vi "TSCAN_GetDllPath.vi"() -> (3 "DllPath":path)   [LabVIEW 2014]
uses:
  Utilities/Global/DLL_Path.vi
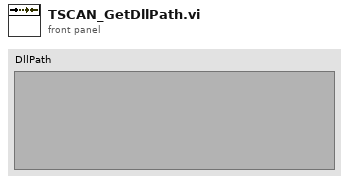
[diagram p1: front panel]
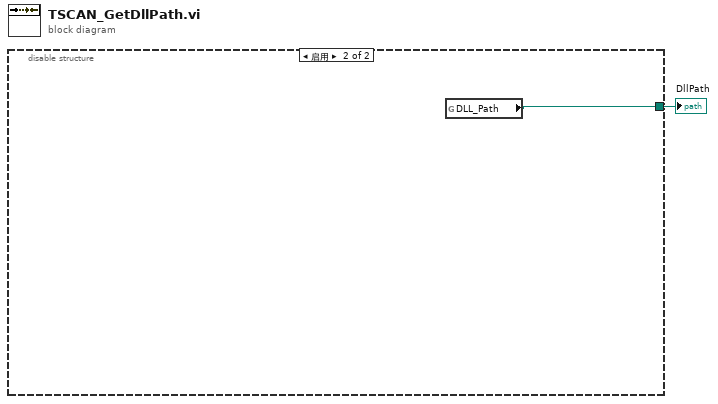
[diagram p0: block diagram]
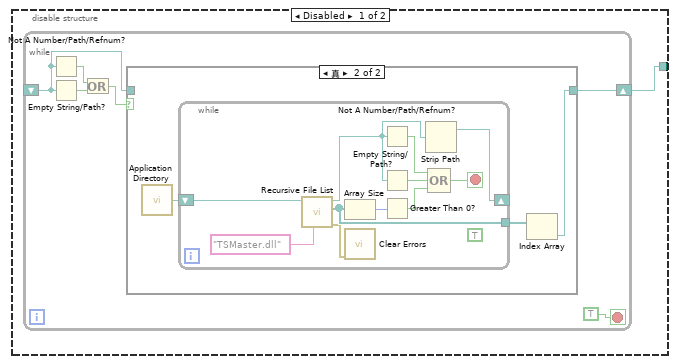
[diagram p2: hidden frame]
diagram:
  n1 = disable-structure shown="启用" {
    disable-tunnel: [w2 w24] -> w1
    frame Disabled {
      n2 = while {
        shift-right: [w8] -> w2
        shift-left: _ -> [w3]
        stop <- TRUE stop-if-true
        n3 = Not A Number/Path/Refnum?(number/path/refnum=w3) -> (NaN/Path/Refnum?=w6:bool)
        n4 = Empty String/Path?(string/path=w3) -> (empty?=w5:bool)
        n5 = Or(x=w6, y=w5) -> (x .or. y?=w4:bool)
        n6 = case shown="真" w4 {
          tunnel: [w9 w12] -> w8
          tunnel: w3 -> [w9 _]
          frame False {
          }
          frame True {
            n7 = call <vilib>:"Application Directory.vi"() -> ("Application Directory"=w10:path)
            n8 = while {
              shift-right: [w15] -> _
              shift-left: w10 -> [w23]
              tunnel: [w14] -> w11
              stop <- w17 stop-if-true
              (unwired) TRUE ("Treat LLBs as Folders?")
              n9 = call <vilib>:"Recursive File List.vi"("pattern"="TSMaster.dll", "Folder Path"=w23) -> ("error out"=w13:errorcluster, "All Files in Dir"=w14:path[], "dup Folder Path"=w16:path)  [unwired: 3 in, 4 out]
              n10 = Array Size(array=w14) -> (size(s)=w21:i32)
              n11 = call <vilib>:"Clear Errors.vi"("error in (no error)"=w13) -> ()  [unwired: 1 in, 6 out]
              n12 = Not A Number/Path/Refnum?(number/path/refnum=w16) -> (NaN/Path/Refnum?=w20:bool)
              n13 = Empty String/Path?(string/path=w16) -> (empty?=w19:bool)
              n14 = Greater Than 0?(x=w21) -> (x > 0?=w18:bool)
              n15 = Strip Path(path=w16) -> (stripped path=w15:path)  [unwired: 1 out]
              n16 = Compound Arithmetic op=OR(w20, w19, w18) -> (w17:bool)
            }
            n17 = Index Array(array=w11) -> (element=w12:path)  [unwired: 1 in]
          }
        }
      }
    }
    frame Enabled {
      n18 = global read "DLL_Path.vi" "DLL_Path"() -> (w24:path)
    }
  }
  "DllPath" <- w1
